vi "ButtonPrototyping.vi"(10 "PrimaryButton":bool) -> ()   [LabVIEW 2024, in "Application.lvclass"]
uses:
  Application.lvclass
  Application.lvclass/Application.ctl
panel:
  out "Boolean 2":bool
  out "Boolean":bool
  in  "SecondaryButton":bool
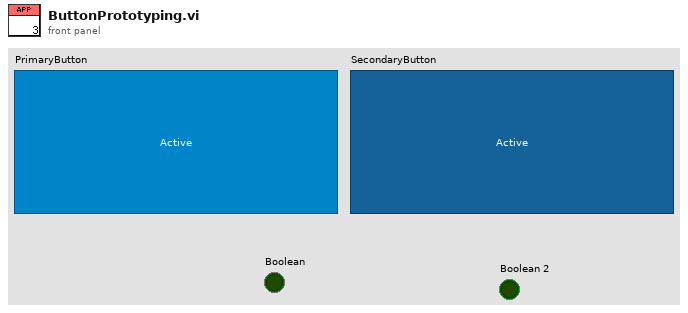
[diagram p1: front panel]
types:
  T1 = cluster{"ActiveBackground":u32, "ActiveBackground":u32}
  T2 = cluster{"PressedBackground":u32, "PressedBackground":u32}
  T3 = cluster{"DisabledBackground":u32, "DisabledBackground":u32}
  T4 = cluster{"DisabledBackground":u32, "DisabledBackground":u32}[]
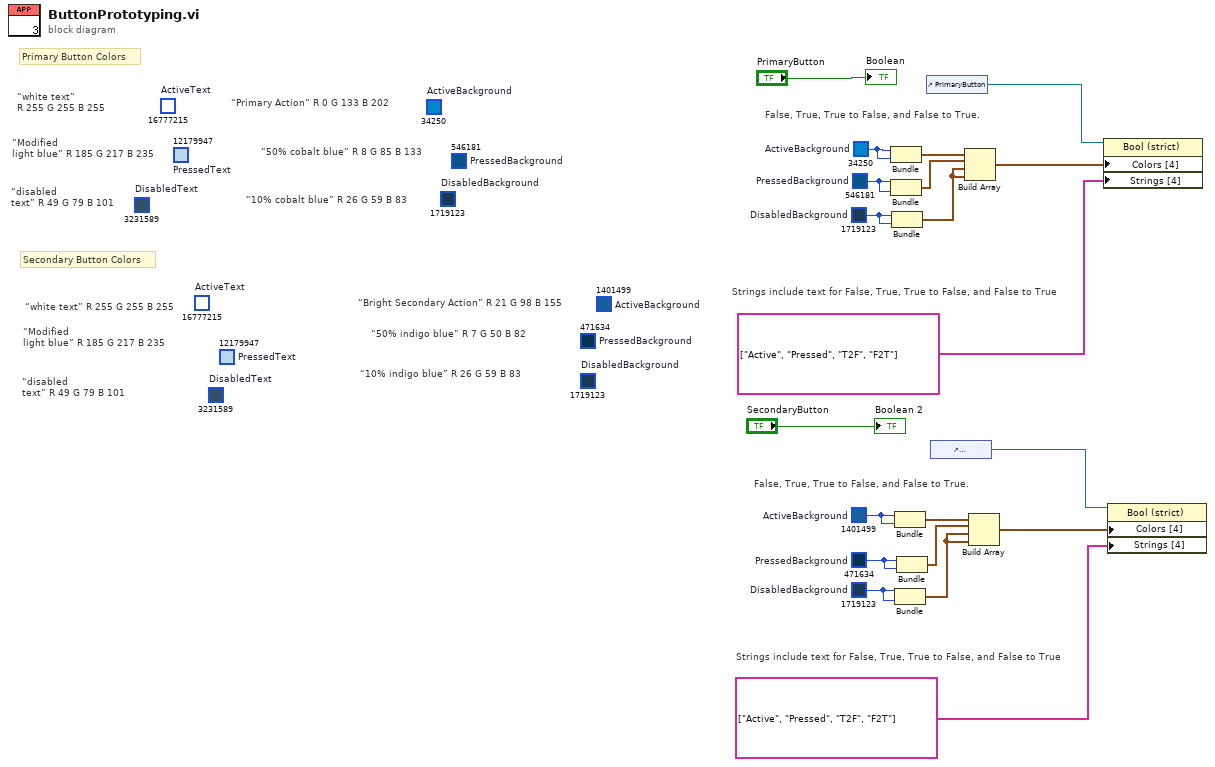
[diagram p0: block diagram]
diagram:
  w5 = u32 1719123  # DisabledBackground
  w6 = u32 471634  # PressedBackground
  w7 = u32 1401499  # ActiveBackground
  (unwired) u32 16777215  # ActiveText
  w18 = u32 546181  # PressedBackground
  w17 = u32 1719123  # DisabledBackground
  w16 = u32 34250  # ActiveBackground
  (unwired) u32 3231589  # DisabledText
  (unwired) u32 12179947  # PressedText
  (unwired) u32 16777215  # ActiveText
  (unwired) u32 1719123  # DisabledBackground
  (unwired) u32 471634  # PressedBackground
  (unwired) u32 1401499  # ActiveBackground
  (unwired) u32 1719123  # DisabledBackground
  (unwired) u32 546181  # PressedBackground
  (unwired) u32 34250  # ActiveBackground
  (unwired) u32 3231589  # DisabledText
  (unwired) u32 12179947  # PressedText
  # "Strings include text for False, True, True to False, and False to True"
  # "False, True, True to False, and False to True."
  # "Strings include text for False, True, True to False, and False to True"
  # "False, True, True to False, and False to True."
  # "Secondary Button Colors"
  # "Primary Button Colors"
  # "“disabled\ntext” R 49 G 79 B 101"
  # "“10% indigo blue” R 26 G 59 B 83"
  # "“Modified\nlight blue” R 185 G 217 B 235"
  # "“50% indigo blue” R 7 G 50 B 82"
  # "“white text” R 255 G 255 B 255"
  # "“Bright Secondary Action” R 21 G 98 B 155"
  # "“10% cobalt blue” R 26 G 59 B 83"
  # "“50% cobalt blue” R 8 G 85 B 133"
  # "“Primary Action” R 0 G 133 B 202"
  # "“disabled\ntext” R 49 G 79 B 101"
  # "“white text”\nR 255 G 255 B 255"
  # "“Modified\nlight blue” R 185 G 217 B 235"
  n1 = Bundle("ActiveBackground"=w16, "ActiveBackground"=w16) -> (w19:T1)  [unwired: 1 in]
  n2 = Bundle("PressedBackground"=w18, "PressedBackground"=w18) -> (w9:T2)  [unwired: 1 in]
  n3 = Bundle("DisabledBackground"=w17, "DisabledBackground"=w17) -> (w8:T3)  [unwired: 1 in]
  n4 = Bundle("ActiveBackground"=w7, "ActiveBackground"=w7) -> (w13:T1)  [unwired: 1 in]
  n5 = Bundle("DisabledBackground"=w5, "DisabledBackground"=w5) -> (w11:T3)  [unwired: 1 in]
  n6 = Bundle("PressedBackground"=w6, "PressedBackground"=w6) -> (w12:T2)  [unwired: 1 in]
  n7 = control-ref of="PrimaryButton"() -> (w15:refnum<vi>)
  n8 = control-ref of="SecondaryButton"() -> (w14:refnum<vi>)
  n9 = Build Array(w19, w9, w8, w8) -> (w20:T4)
  n10 = Build Array(w13, w12, w11, w11) -> (w10:T4)
  n11 = property class="Bool (strict)"(reference=w15, "Colors [4]"=w20, "Strings [4]"=string[] ["Active", "Pressed", "T2F", "F2T"]) -> ()  [unwired: 1 in, 2 out]
  n12 = property class="Bool (strict)"(reference=w14, "Colors [4]"=w10, "Strings [4]"=string[] ["Active", "Pressed", "T2F", "F2T"]) -> ()  [unwired: 1 in, 2 out]
  "Boolean" <- "PrimaryButton"
  "Boolean 2" <- "SecondaryButton"
